vi "VI-Rename Dependencies.vi"(0 "VIref in":refnum<vi>, 5 "Old prefix":string="EPT", 7 "New prefix":string, 9 "Icon Template":refnum<class "Icon Framework.lvclass">, 11 "error in (no error)":errorcluster) -> (4 "VIref out":refnum<vi>, 15 "error out":errorcluster)   [LabVIEW 2020]
uses:
  <vilib>/LabVIEW Icon API/lv_icon/Classes/Icon Framework/Icon Framework.lvclass
  <vilib>/regexp/Match Regular Expression.xnode
  <vilib>/LabVIEW Icon API/lv_icon/Classes/Icon/Icon.lvclass
  <vilib>/LabVIEW Icon API/LabVIEW Icon API.lvlib
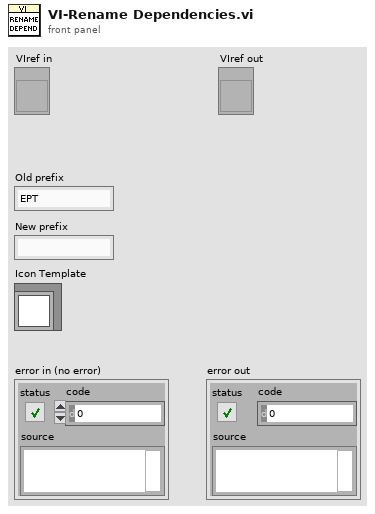
[diagram p1: front panel]
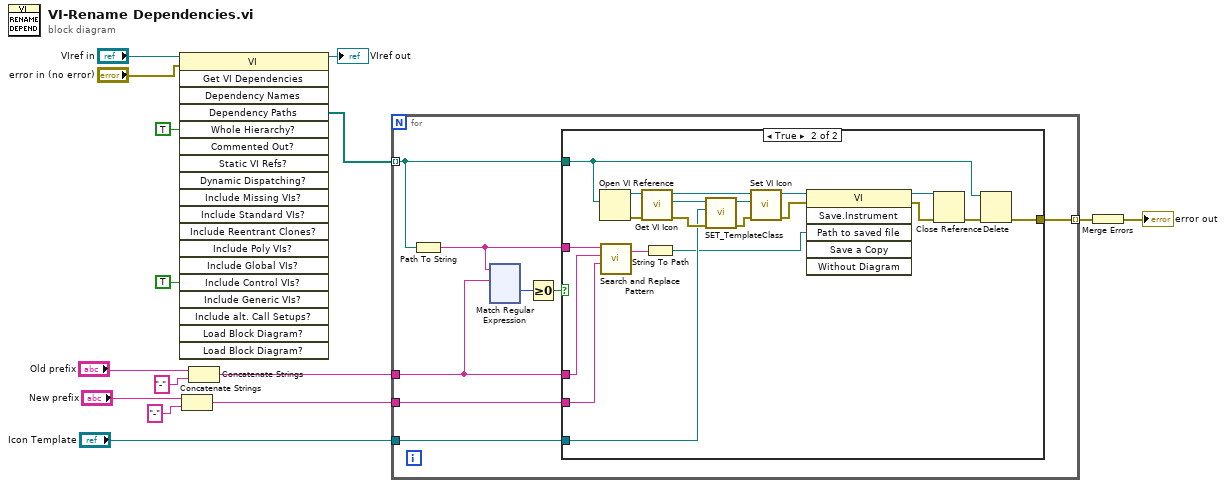
[diagram p0: block diagram]
diagram:
  n1 = invoke class="VI" method="Get VI Dependencies"(reference="VIref in", error in="error in (no error)", "Whole Hierarchy?"=TRUE, "Include Control VIs?"=TRUE) -> (reference out=→"VIref out":refnum<vi>, "Dependency Paths"=w15:path[])  [unwired: 15 in, 17 out]
  n2 = Concatenate Strings("New prefix", "-") -> (w8:string)
  n3 = Concatenate Strings("Old prefix", "-") -> (w7:string)
  n4 = for {
    tunnel: w15 -> [w22] mode=indexing
    tunnel: [w23] -> w6 mode=indexing
    tunnel: w8 -> [w17]
    tunnel: w7 -> [w18]
    tunnel: "Icon Template" -> [w16]
    n5 = Path To String(path=w22) -> (string=w19:string)
    n6 = xnode "Match Regular Expression"("input string"=w19, "regular expression"=w18) -> ("offset past match"=w21:i32)  [unwired: 4 in, 4 out]
    n7 = Greater Or Equal To 0?(x=w21) -> (x >= 0?=w20:bool)
    n8 = case shown="True" w20 {
      tunnel: w22 -> [_ w154]
      tunnel: [_ w153] -> w23
      tunnel: w19 -> [_ w152]
      tunnel: w18 -> [_ w151]
      tunnel: w17 -> [_ w150]
      tunnel: w16 -> [_ w143]
      frame False {
      }
      frame True {
        n9 = Open VI Reference(vi path=w154) -> (vi reference=w146:refnum<vi>, error out=w145:errorcluster)  [unwired: 5 in]
        n10 = call <vilib>:"Search and Replace Pattern.vi"("string"=w152, "regular expression (\"\")"=w151, "replace string (\"\")"=w150) -> ("result string"=w149:string)  [unwired: 2 in, 1 out]
        n11 = call <vilib>:"Get VI Icon.vi"("error in (no error)"=w145, "VI Refnum in"=w146) -> ("error out"=w144:errorcluster, "Icon"=w141:refnum<class "Icon.lvclass">, "VI Refnum out"=w142:refnum<vi>)  [unwired: 7 in]
        n12 = String To Path(string=w149) -> (path=w138:path)
        n13 = call-dynamic "SET_TemplateClass.vi"("error in (no error)"=w144, "Icon Framework.lvclass"=w143, "Icon.lvclass in"=w141) -> ("error out"=w140:errorcluster, "Icon.lvclass out"=w139:refnum<class "Icon.lvclass">)  [unwired: 7 in]
        n14 = call <vilib>:"Set VI Icon.vi"("error in (no error)"=w140, "Icon"=w139, "VI Refnum in"=w142) -> ("error out"=w148:errorcluster, "VI Refnum out"=w147:refnum<vi>)  [unwired: 7 in]
        n15 = invoke class="VI" method="Save.Instrument"(reference=w147, error in=w148, "Path to saved file"=w138) -> (reference out=w156:refnum<vi>, error out=w157:errorcluster)  [unwired: 3 in, 4 out]
        n16 = Close Reference(reference=w156, error in (no error)=w157) -> (error out=w155:errorcluster)
        n17 = Delete(path (use dialog)=w154, error in=w155) -> (error out=w153:errorcluster)  [unwired: 3 in, 2 out]
      }
    }
  }
  n18 = Merge Errors(w6) -> (→"error out":errorcluster)
